vi "XY Chart Buffer_PINK.vi"(8 "clear first (no:F)":bool, 9 "chart length (points)":i32=100, 10 "YNew":dbl, 11 "XNew":dbl) -> (1 "Value Y":dbl[](array[numeric]), 3 "Value X":dbl[](array[numeric]))   [LabVIEW 2023]
doc: "This reentrant VI uses an XY graph to mimic the behavior of an XY chart, in that it plots a stipulated amount of the most recently acquired data points. The chart data is stored in a static local variable of the output XY chart indicator.\n\nBecause the VI has been marked reentrant (in VI setup), you can make multiple parallel calls to the VI without confusing the memory. Use the new points array input to supply multiple points at once, or leave the array unwired (empty) and use the new point cluster input to supply one point at a time. If the locally stored chart array is not equal to chart length, it is expanded to that lenght by replicating the most recently acquired point. Data in excess of the history length is discarded. Set clear first to clear the chart history before processing the new points."
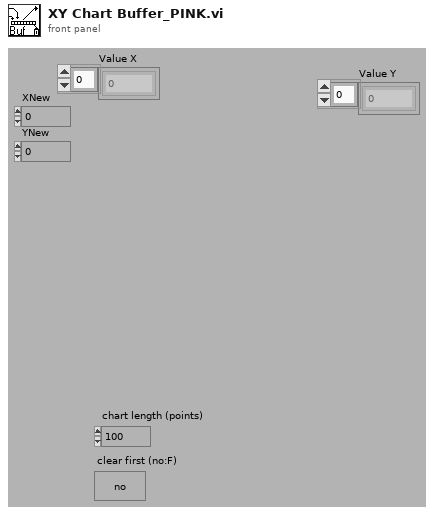
[diagram p1: front panel]
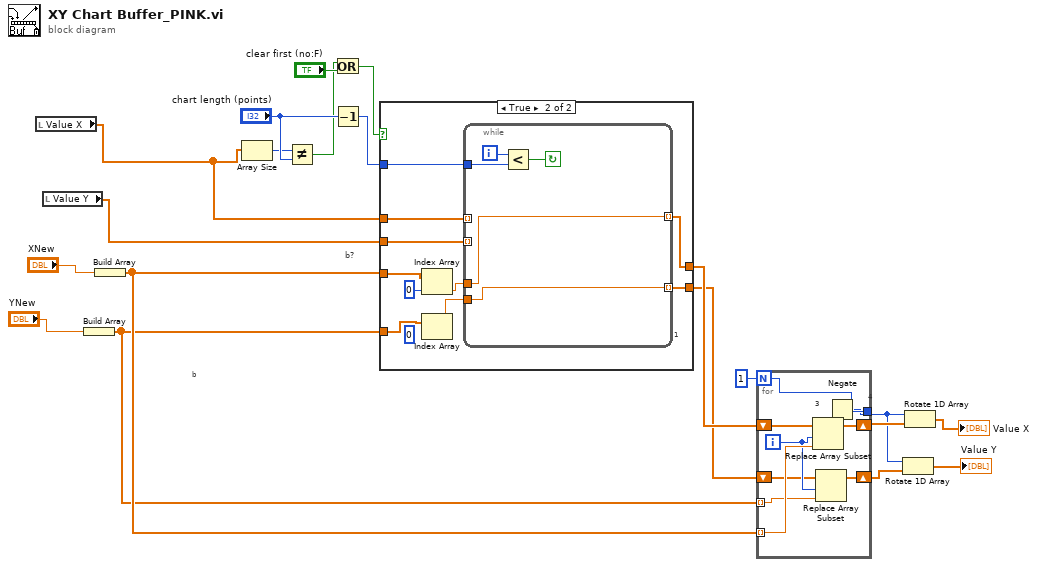
[diagram p0: block diagram]
diagram:
  # "4"
  # "1"
  # "b"
  # "b?"
  n1 = local read "Value X"() -> (w2:dbl[])
  n2 = local read "Value Y"() -> (w1:dbl[])
  n3 = Build Array("YNew") -> (w4:dbl[])
  n4 = Build Array("XNew") -> (w5:dbl[])
  n5 = Array Size(array=w2) -> (size(s)=w18:i32)
  n6 = Not Equal?(x=w18, y="chart length (points)") -> (x != y?=w15:bool)
  n7 = Or(x=w15, y="clear first (no:F)") -> (x .or. y?=w14:bool)
  n8 = Decrement(x="chart length (points)") -> (x-1=w13:i32)
  n9 = case shown="True" w14 {
    tunnel: [w23 w25] -> w19
    tunnel: w13 -> [_ w33]
    tunnel: w5 -> [_ w30]
    tunnel: w4 -> [_ w29]
    tunnel: [w22 w27] -> w3
    tunnel: w2 -> [w23 w26]
    tunnel: w1 -> [w22 w24]
    frame False {
    }
    frame True {
      (unwired) 0
      n10 = Index Array(array=w30, index=0) -> (element=w31:dbl)
      n11 = Index Array(array=w29) -> (element=w28:dbl)  [unwired: 1 in]
      n12 = while {
        tunnel: w31 -> [w35]
        tunnel: w33 -> [w38]
        tunnel: w28 -> [w34]
        tunnel: [w34] -> w27 mode=indexing
        tunnel: w26 -> [_] mode=indexing
        tunnel: [w35] -> w25 mode=indexing
        tunnel: w24 -> [_] mode=indexing
        i -> [w37]
        stop <- w36 continue-if-true
        n13 = Less?(x=w37, y=w38) -> (x < y?=w36:bool)
      }
    }
  }
  n14 = for {
    N: 1 -> [w44]
    shift-right: [w46] -> w21
    shift-left: w19 -> [w45]
    tunnel: w5 -> [w43] mode=indexing
    tunnel: [w44] -> w17
    shift-right: [w40] -> w8
    shift-left: w3 -> [w41]
    tunnel: w4 -> [w39] mode=indexing
    i -> [w42]
    # "3"
    n15 = Replace Array Subset(array=w45, new element=w43, index=w42) -> (w46:dbl[])
    n16 = Replace Array Subset(array=w41, new element=w39, index=w42) -> (w40:dbl[])
  }
  n17 = Negate(x=w17) -> (-x=w9:i32)
  n18 = Rotate 1D Array(1:w8, 2:w9) -> (0:→"Value Y":dbl[])
  n19 = Rotate 1D Array(1:w21, 2:w9) -> (0:→"Value X":dbl[])
